vi "Outer Measure.vi"(8 "error in (no error)":errorcluster, 11 "Measurement3D in":refnum<class "Measurement3D.lvclass">) -> (0 "error out":errorcluster, 2 "Current Value":dbl, 3 "Measurement3D out":refnum<class "Measurement3D.lvclass">)   [LabVIEW 2014, in "Measurement3D.lvclass"]
uses:
  Measurement3D.lvclass
  Instrument/Instrument/Instrument.lvclass
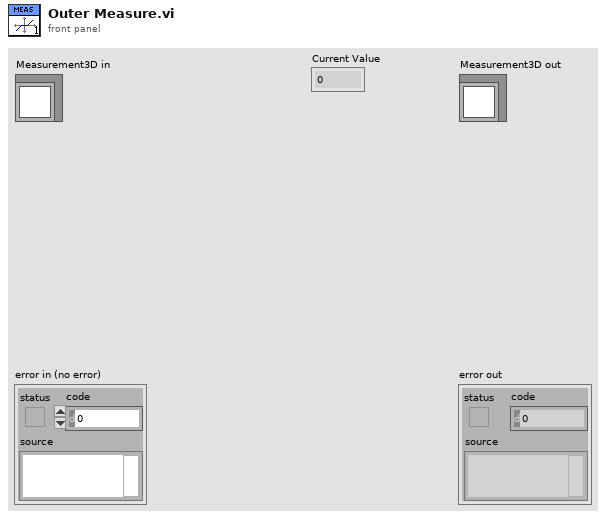
[diagram p1: front panel]
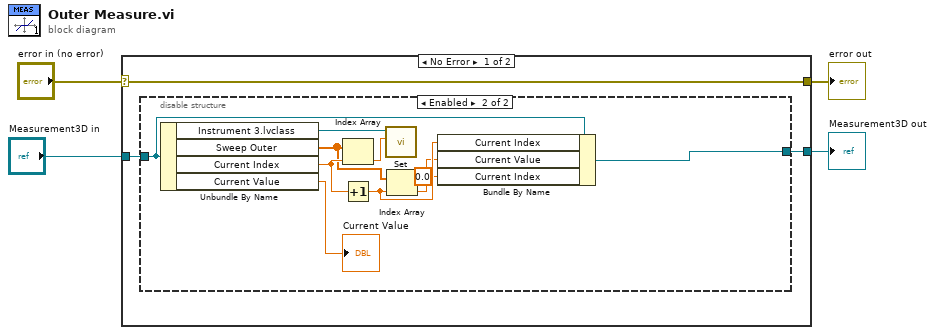
[diagram p0: block diagram]
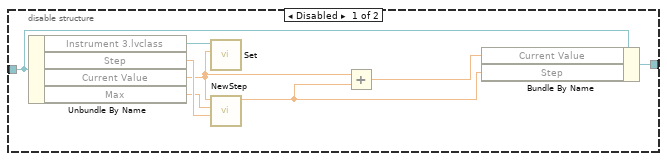
[diagram p2: hidden frame]
diagram:
  n1 = case shown="No Error" "error in (no error)" {
    selector: "error in (no error)" -> [w7 w27]
    tunnel: [w7 w27] -> w3
    tunnel: [w5 w26] -> w1
    tunnel: "Measurement3D in" -> [w6 w26]
    frame No Error {
      n2 = disable-structure shown="Enabled" {
        disable-tunnel: w6 -> [w9 w23]
        disable-tunnel: [w8 w17] -> w5
        frame Disabled {
          n3 = Unbundle By Name(w9) -> ("Instrument 3.lvclass"=w15:refnum<class "Instrument.lvclass">, "Step"=w14:dbl, "Current Value"=w12:dbl, "Max"=w13:dbl)
          n4 = call-dynamic "Set.vi"("Numeric"=w12, "Instrument in"=w15) -> ()  [unwired: 8 in, 2 out]
          n5 = call "NewStep.vi"("Step"=w14, "Max"=w13, "Current Value"=w12) -> ("Step 2"=w10:dbl)  [unwired: 8 in]
          n6 = Add(x=w12, y=w10) -> (x+y=w11:dbl)
          n7 = Bundle By Name(cluster=w9, "Current Value"=w11, "Step"=w10) -> (w8:refnum<class "Measurement3D.lvclass">)
        }
        frame Enabled {
          n8 = Unbundle By Name(w23) -> ("Instrument 3.lvclass"=w25:refnum<class "Instrument.lvclass">, "Sweep Outer"=w21:dbl[], "Current Index"=w22:dbl, "Current Value"=→"Current Value":dbl)
          n9 = Index Array(array=w21, index=w22) -> (element=w24:dbl)
          n10 = Increment(x=w22) -> (x+1=w20:dbl)
          n11 = call-dynamic "Set.vi"("Numeric"=w24, "Instrument in"=w25) -> ()  [unwired: 8 in, 2 out]
          n12 = Index Array(array=w21, index=w20) -> (element=w19:dbl)
          n13 = Bundle By Name(cluster=w23, "Current Index"=w20, "Current Value"=w19, "Current Index"=0.0 ("Inner Loop.Current Index")) -> (w17:refnum<class "Measurement3D.lvclass">)
        }
      }
    }
    frame Error {
    }
  }
  "error out" <- w3
  "Measurement3D out" <- w1
